vi "FileOnController.vi"(8 "error in (no error)":errorcluster, 9 "Silent?":bool, 10 "(Empty=No Action)":path caption="File Path & Name", 11 "controller in":refnum<k24>) -> (0 "error out":errorcluster, 2 "File Exist?":bool, 3 "controller out":refnum<k24>)   [LabVIEW 2010]
uses:
  c:/aerotech/controller/5.xx.xxx/ensemble/pc/labview/2010/bin/Aerotech.Ensemble.dll
  bin/Aerotech.Ensemble.dll
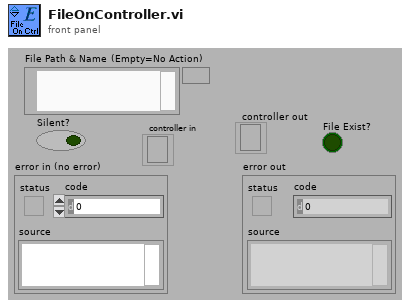
[diagram p1: front panel]
types:
  T1 = cluster{"Name":string, "CreationTime":timestamp, "Size":i32, "UserAttributes":i32, "SystemAttributes":i32}[]
  T2 = cluster{"Name":string, "CreationTime":timestamp, "Size":i32, "UserAttributes":i32, "SystemAttributes":i32}
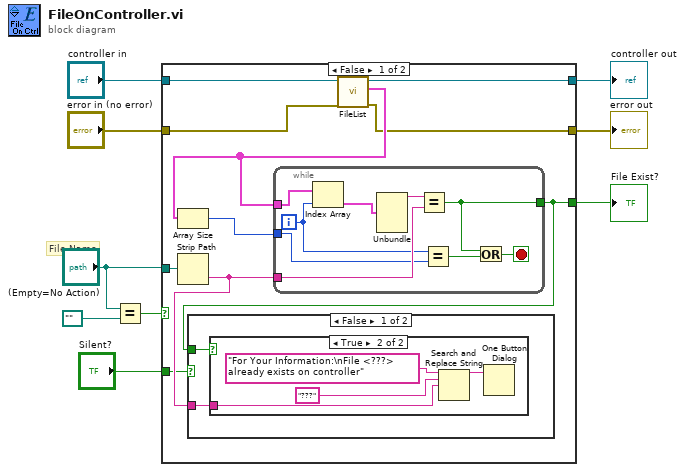
[diagram p0: block diagram]
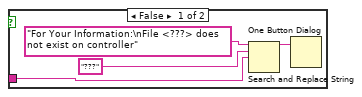
[diagram p2: hidden frame]
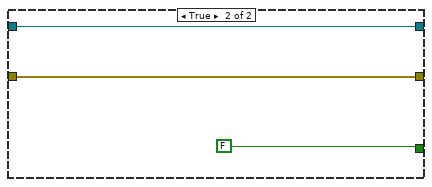
[diagram p4: hidden frame]
diagram:
  # "File Name"
  n1 = Equal?(x="(Empty=No Action)", y=path "" ("x")) -> (x = y?=w9:bool)
  n2 = case shown="False" w9 {
    tunnel: "(Empty=No Action)" -> [w18 _]
    tunnel: [w15 FALSE] -> w6
    tunnel: [w14 w40] -> w5
    tunnel: [w13 w41] -> w4
    tunnel: "controller in" -> [w12 w41]
    tunnel: "error in (no error)" -> [w11 w40]
    tunnel: "Silent?" -> [w10 _]
    frame False {
      n3 = Strip Path(path=w18) -> (name=w17:string)  [unwired: 1 out]
      n4 = call "FileList.vi"("error in (no error)"=w11, "controller in"=w12) -> ("error out"=w14:errorcluster, "File List"=w19:T1, "controller out"=w13:refnum<k24>)  [unwired: 6 in, 1 out]
      n5 = Array Size(array=w19) -> (size(s)=w16:i32)
      n6 = while {
        tunnel: w19 -> [w28]
        tunnel: w17 -> [w25]
        tunnel: [w21] -> w15
        tunnel: w16 -> [w23]
        i -> [w24]
        stop <- w22 stop-if-true
        n7 = Index Array(array=w28, index=w24) -> (element=w27:T2)
        n8 = Unbundle(w27) -> ("Name"=w26:string)  [unwired: 4 out]
        n9 = Equal?(x=w26, y=w25) -> (x = y?=w21:bool)
        n10 = Equal?(x=w24, y=w23) -> (x = y?=w20:bool)
        n11 = Or(x=w21, y=w20) -> (x .or. y?=w22:bool)
      }
      n12 = case shown="False" w10 {
        tunnel: w15 -> [w30 _]
        tunnel: w17 -> [w29 _]
        frame False {
          n13 = case shown="True" w30 {
            tunnel: w29 -> [w31 w35]
            frame False {
              n14 = Search and Replace String(input string="For Your Information:\nFile <???> does not exist on controller" ("message"), search string="???", replace string=w31) -> (result string=w34:string)  [unwired: 5 in, 3 out]
              n15 = One Button Dialog(message=w34) -> ()  [unwired: 1 in, 1 out]
            }
            frame True {
              n16 = Search and Replace String(input string="For Your Information:\nFile <???> already exists on controller" ("message"), search string="???", replace string=w35) -> (result string=w36:string)  [unwired: 5 in, 3 out]
              n17 = One Button Dialog(message=w36) -> ()  [unwired: 1 in, 1 out]
            }
          }
        }
        frame True {
        }
      }
    }
    frame True {
    }
  }
  "controller out" <- w4
  "error out" <- w5
  "File Exist?" <- w6
